vi "Read Consumer Name.vi"(8 "error in (no error)":errorcluster, 11 "Reflected Name Consumer in":refnum<class "Test Consumer.lvclass">) -> (0 "error out":errorcluster, 2 "Reflected Name":string, 3 "Reflected Name Consumer out":refnum<class "Test Consumer.lvclass">)   [LabVIEW 2027, in "Test Consumer.lvclass"]
uses:
  Test Consumer.lvclass
  Test Consumer.lvclass/Test Consumer.ctl
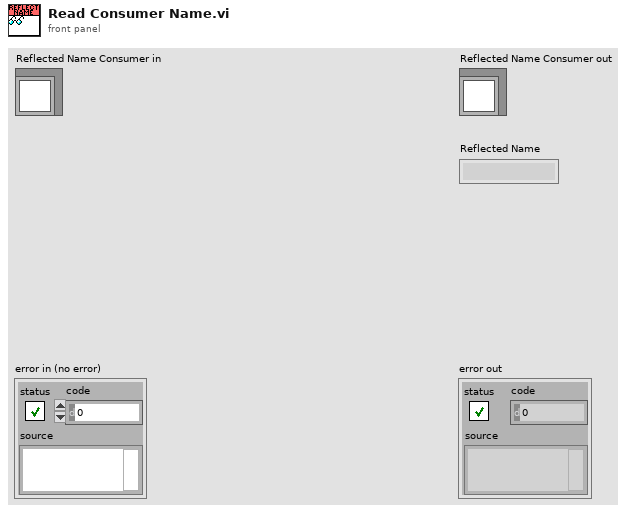
[diagram p1: front panel]
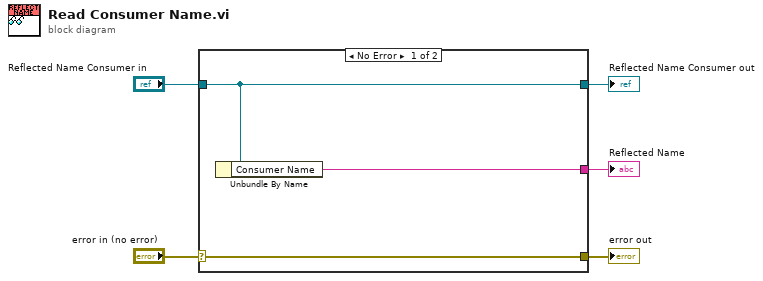
[diagram p0: block diagram]
diagram:
  n1 = case shown="No Error" "error in (no error)" {
    selector: "error in (no error)" -> [w8 w9]
    tunnel: [w8 w9] -> w4
    tunnel: [w7 w10] -> w2
    tunnel: "Reflected Name Consumer in" -> [w7 w10]
    tunnel: [w6 _] -> w1
    frame No Error {
      n2 = Unbundle By Name(w7) -> ("Consumer Name"=w6:string)
    }
    frame Error {
    }
  }
  "error out" <- w4
  "Reflected Name Consumer out" <- w2
  "Reflected Name" <- w1
